vi "subVI_YPID.vi"(8 "Cumulative Error In":dbl=0.39154375000000835, 9 "Previous Error":dbl=7.812499999992895e-05, 10 "Encoder Position [mm]":dbl=0.99984375, 11 "Desired Position [mm]":dbl=1.0) -> (0 "Cumulative Error Out":dbl=0.39154531250000835, 1 "Error":dbl=0.00015624999999996891, 3 "Control Signal [V]":dbl=-0.939201562500288)   [LabVIEW 2017]
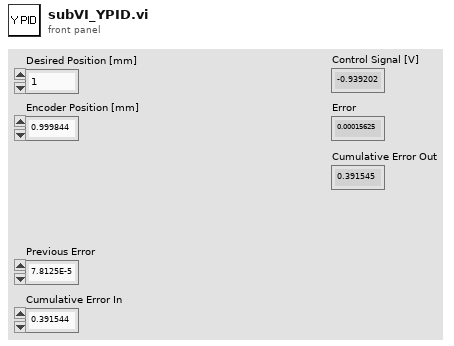
[diagram p1: front panel]
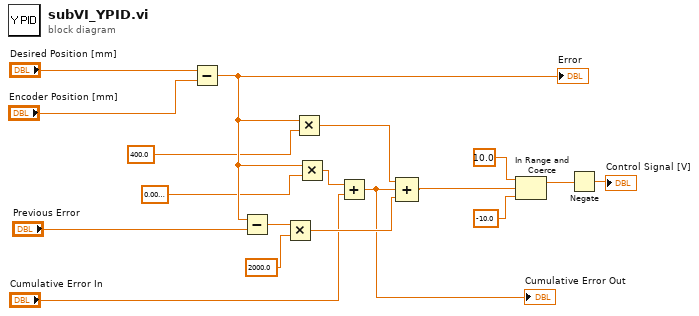
[diagram p0: block diagram]
diagram:
  n1 = Subtract(x="Desired Position [mm]", y="Encoder Position [mm]") -> (x-y=w16:dbl)
  "Error" <- w16
  n2 = Subtract(x=w16, y="Previous Error") -> (x-y=w14:dbl)
  n3 = Multiply(x=w14, y=2000.0 ("yd")) -> (x*y=w12:dbl)
  n4 = Multiply(x=w16, y=400.0 ("yp")) -> (x*y=w13:dbl)
  n5 = Multiply(x=w16, y=0.009999999999999997 ("yi")) -> (x*y=w11:dbl)
  n6 = Add(x=w11, y="Cumulative Error In") -> (x+y=w7:dbl)
  "Cumulative Error Out" <- w7
  n7 = Compound Arithmetic op=ADD(w13, w7, w12) -> (w3:dbl)
  n8 = In Range and Coerce(upper limit=10.0, x=w3, lower limit=-10.0) -> (coerced(x)=w1:dbl)  [unwired: 1 out]
  n9 = Negate(x=w1) -> (-x=→"Control Signal [V]":dbl)
